vi "ejemplo.vi"(8 "error in (no error)":errorcluster, 11 "Class 2 in":refnum<class "Class 2.lvclass">) -> (0 "error out":errorcluster)   [LabVIEW 2019, in "Class 2.lvclass"]
uses:
  Class 2.lvclass
  Class 2.lvclass/Class 2.ctl
panel:
  out "Boolean 2":bool
  out "Boolean":bool
  in  "s":bool
  in  "stop":bool
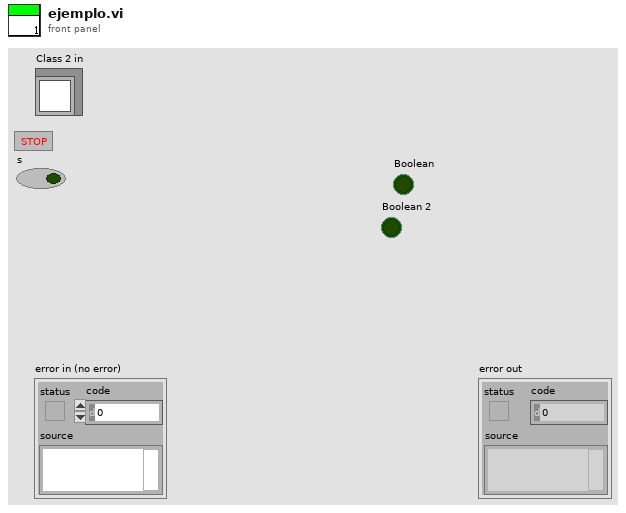
[diagram p1: front panel]
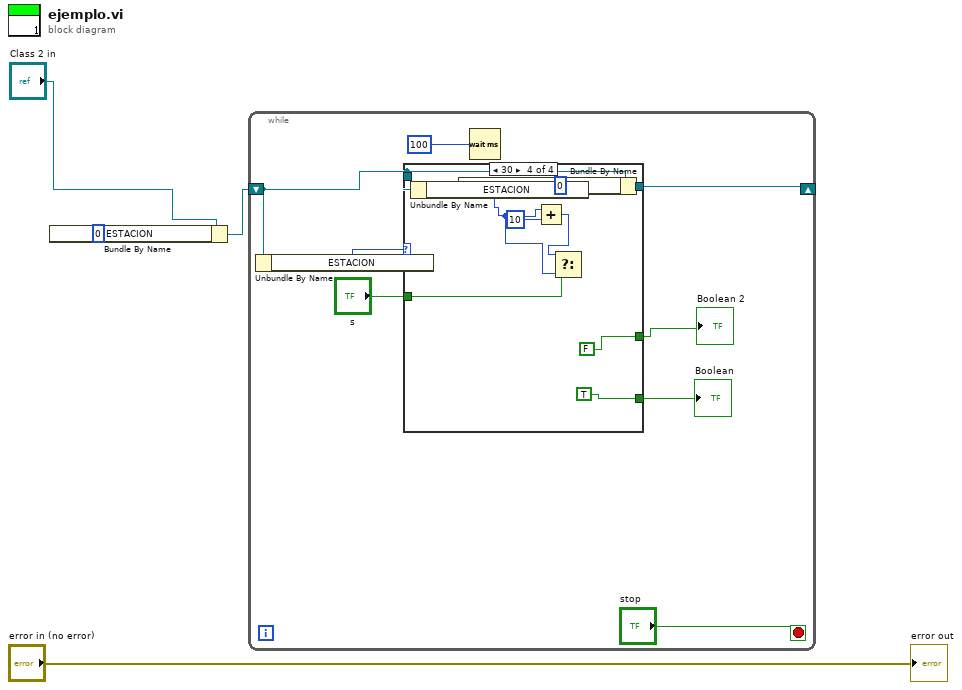
[diagram p0: block diagram]
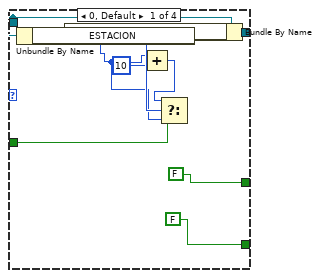
[diagram p2: hidden frame]
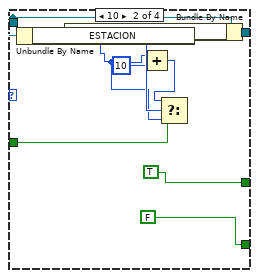
[diagram p3: hidden frame]
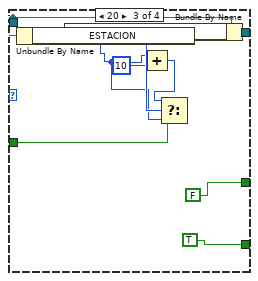
[diagram p4: hidden frame]
diagram:
  n1 = Bundle By Name(cluster="Class 2 in", "ESTACION"=0 ("State")) -> (w2:refnum<class "Class 2.lvclass">)
  n2 = while {
    shift-right: [w11] -> _
    shift-left: w2 -> [w8]
    stop <- "stop" stop-if-true
    n3 = Unbundle By Name(w8) -> ("ESTACION"=w7:i32)
    n4 = case shown="30" w7 {
      tunnel: w8 -> [w21 w30 w39 w48]
      tunnel: [w20 w29 w38 w47] -> w11
      tunnel: "s" -> [w18 w27 w36 w46]
      tunnel: [FALSE ("Boolean 2") FALSE ("Boolean 2") TRUE ("Boolean 2") TRUE ("Boolean 2")] -> w6
      tunnel: [FALSE ("Boolean 2") TRUE ("Boolean 2") FALSE ("Boolean 2") FALSE ("Boolean 2")] -> w5
      frame 0, Default {
        n5 = Unbundle By Name(w21) -> ("ESTACION"=w17:i32)
        n6 = Add(x=w17, y=10) -> (x+y=w15:i32)
        n7 = Select(t=w15, s=w18, f=w17) -> (s? t:f=w19:i32)
        n8 = Bundle By Name(cluster=w21, "ESTACION"=w19) -> (w20:refnum<class "Class 2.lvclass">)
      }
      frame 10 {
        n9 = Unbundle By Name(w30) -> ("ESTACION"=w26:i32)
        n10 = Add(x=w26, y=10) -> (x+y=w24:i32)
        n11 = Select(t=w24, s=w27, f=w26) -> (s? t:f=w28:i32)
        n12 = Bundle By Name(cluster=w30, "ESTACION"=w28) -> (w29:refnum<class "Class 2.lvclass">)
      }
      frame 20 {
        n13 = Unbundle By Name(w39) -> ("ESTACION"=w35:i32)
        n14 = Add(x=w35, y=10) -> (x+y=w33:i32)
        n15 = Select(t=w33, s=w36, f=w35) -> (s? t:f=w37:i32)
        n16 = Bundle By Name(cluster=w39, "ESTACION"=w37) -> (w38:refnum<class "Class 2.lvclass">)
      }
      frame 30 {
        n17 = Unbundle By Name(w48) -> ("ESTACION"=w45:i32)
        n18 = Bundle By Name(cluster=w48, "ESTACION"=0 ("State")) -> (w47:refnum<class "Class 2.lvclass">)
        n19 = Add(x=w45, y=10) -> (x+y=w43:i32)
        n20 = Select(t=w43, s=w46, f=w45) -> ()  [unwired: 1 out]
      }
    }
    "Boolean" <- w6
    "Boolean 2" <- w5
    n21 = Wait (ms)(milliseconds to wait=u32 100) -> ()  [unwired: 1 out]
  }
  "error out" <- "error in (no error)"
